vi "LKS 340 check temp stability.vi"(0 "Set point proximity":dbl=0.05 format="%.3f", 1 "Stability":dbl=0.05 format="%.3f", 2 "GPIB Address":dbl=12.0, 3 "seconds to wait":u32=30, 4 "error in":errorcluster) -> (7 "error out":errorcluster)   [LabVIEW 2014]
panel:
  out "Temperature":dbl=26.719 format="%.4f"
  out "Waveform Chart":dbl(graph)=26.719
  out "Set Point":dbl=40.0 format="%.4f"
  in  "Sample time Secs":dbl=1.0
  # "Checking for temperature stability"
  # "Temperature must be within +/-"
  # "of set point"
  # "and stable within +/-"
  # "over"
  # "Seconds"
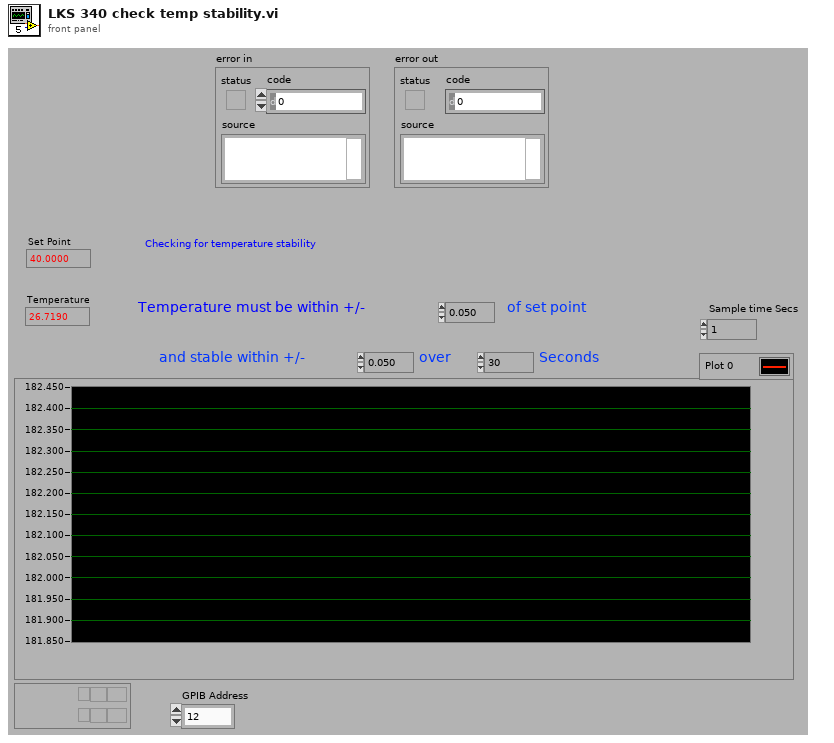
[diagram p1: front panel]
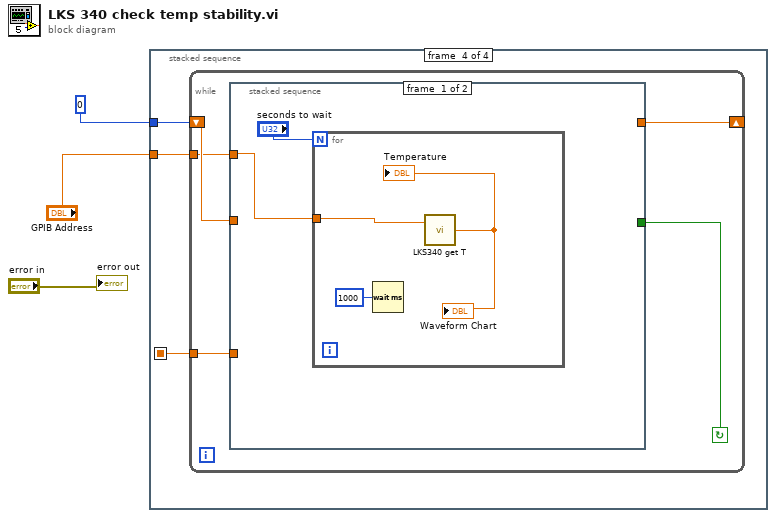
[diagram p0: block diagram]
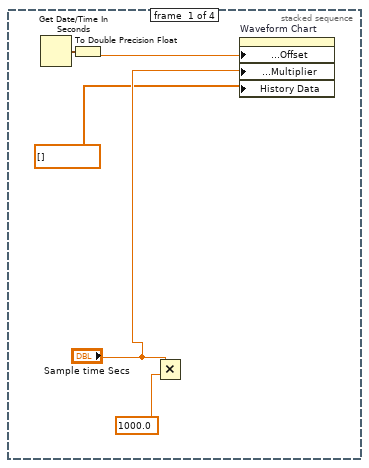
[diagram p2: hidden frame]
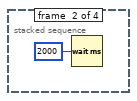
[diagram p3: hidden frame]
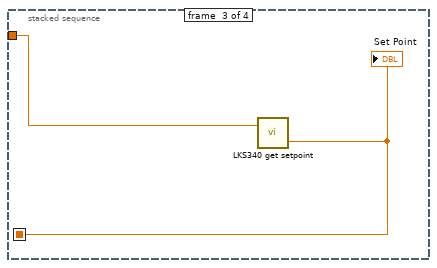
[diagram p4: hidden frame]
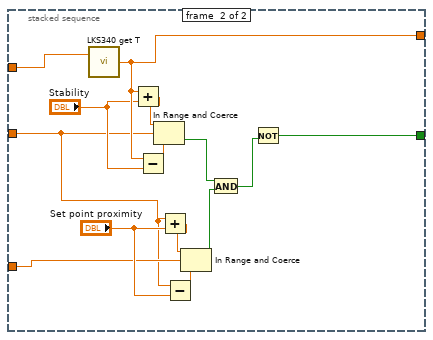
[diagram p5: hidden frame]
diagram:
  n1 = stacked-sequence {
    seq-local: [_ _ w10 _] -> [_ _ _ w12]
    tunnel: 0 -> [_ _ _ w14]
    tunnel: "GPIB Address" -> [_ _ w11 w13]
    frame #0 {
      n2 = Get Date/Time In Seconds() -> (seconds since 1Jan1904=w4:timestamp)
      n3 = To Double Precision Float(number=w4) -> (double precision float=w7:dbl)
      n4 = Multiply(x="Sample time Secs", y=1000.0) -> ()  [unwired: 1 out]
      n5 = property on="Waveform Chart" class="WFChart (strict)"("X Scale.Offset and Multiplier:Offset"=w7, "X Scale.Offset and Multiplier:Multiplier"="Sample time Secs", "History Data"=dbl[] [] ("Write Attribute")) -> ()  [unwired: 2 in, 2 out]
    }
    frame #1 {
      n6 = Wait (ms)(milliseconds to wait=u32 2000) -> ()  [unwired: 1 out]
    }
    frame #2 {
      n7 = call "LKS340 get setpoint.vi"("GPIB Adress"=w11) -> ("Set Point"=w10:dbl)  [unwired: 2 in]
      "Set Point" <- w10
    }
    frame #3 {
      n8 = while {
        tunnel: w12 -> [w15]
        tunnel: w13 -> [w16]
        shift-left: w14 -> [w17]
        shift-right: [w18] -> _
        stop <- w19 continue-if-true
        n9 = stacked-sequence {
          tunnel: [_ w36] -> w19
          tunnel: [_ w35] -> w18
          tunnel: w17 -> [_ w25]
          tunnel: w16 -> [w20 w33]
          tunnel: w15 -> [_ w26]
          frame #0 {
            n10 = for {
              N: "seconds to wait" -> [_]
              tunnel: w20 -> [w22]
              n11 = Wait (ms)(milliseconds to wait=u32 1000) -> ()  [unwired: 1 out]
              n12 = call "LKS340 get T.vi"("GPIB Adress"=w22) -> ("Temperature"=→"Temperature" →"Waveform Chart":dbl)  [unwired: 3 in]
            }
          }
          frame #1 {
            n13 = call "LKS340 get T.vi"("GPIB Adress"=w33) -> ("Temperature"=w35:dbl)  [unwired: 3 in]
            n14 = Add(x=w35, y="Stability") -> (x+y=w38:dbl)
            n15 = Subtract(x=w35, y="Stability") -> (x-y=w37:dbl)
            n16 = In Range and Coerce(upper limit=w38, x=w25, lower limit=w37) -> (In Range?=w28:bool)  [unwired: 1 out]
            n17 = Add(x=w25, y="Set point proximity") -> (x+y=w32:dbl)
            n18 = Subtract(x=w25, y="Set point proximity") -> (x-y=w31:dbl)
            n19 = In Range and Coerce(upper limit=w32, x=w26, lower limit=w31) -> (In Range?=w30:bool)  [unwired: 1 out]
            n20 = And(x=w28, y=w30) -> (x .and. y?=w27:bool)
            n21 = Not(x=w27) -> (.not. x?=w36:bool)
          }
        }
      }
    }
  }
  "error out" <- "error in"
